vi "PCert-ConfigPageNF-AskDB.vi"(6 "Timeout":i32=100 format="%dmsec", 8 "error in (no error)":errorcluster, 9 "Request Body":string, 10 "Request Header":string, 11 "ERP-ConfigPageNF in":refnum<class "PCert-ConfigPageNF.lvclass">) -> (0 "error out":errorcluster, 2 "Ask Operation Failed":bool, 3 "ERP-ConfigPageNF out":refnum<class "PCert-ConfigPageNF.lvclass">, 5 "Raw Column Data From DB":string[](array[string]), 7 "Raw Data From DB":string[][](array[string]))   [LabVIEW 2013, in "PCert-ConfigPageNF.lvclass"]
uses:
  PCert-ConfigPageNF.lvclass
  PCert-ConfigPageNF.lvclass/PCert-ConfigPageNF.ctl
  ftw-dataflow/Actor/src/Connector/FTW-ActorConnector.lvclass
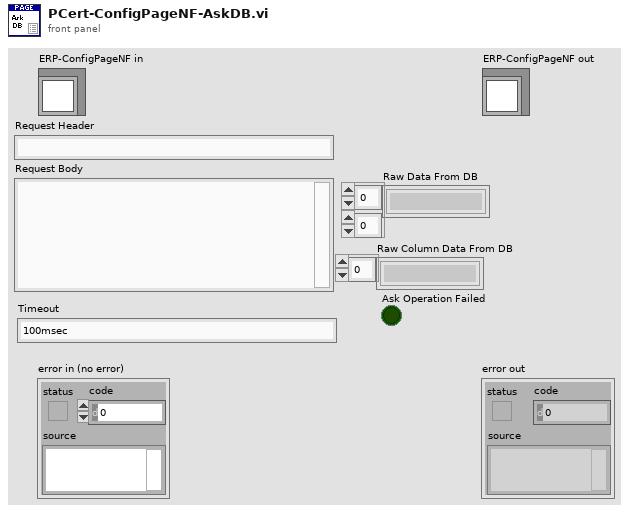
[diagram p1: front panel]
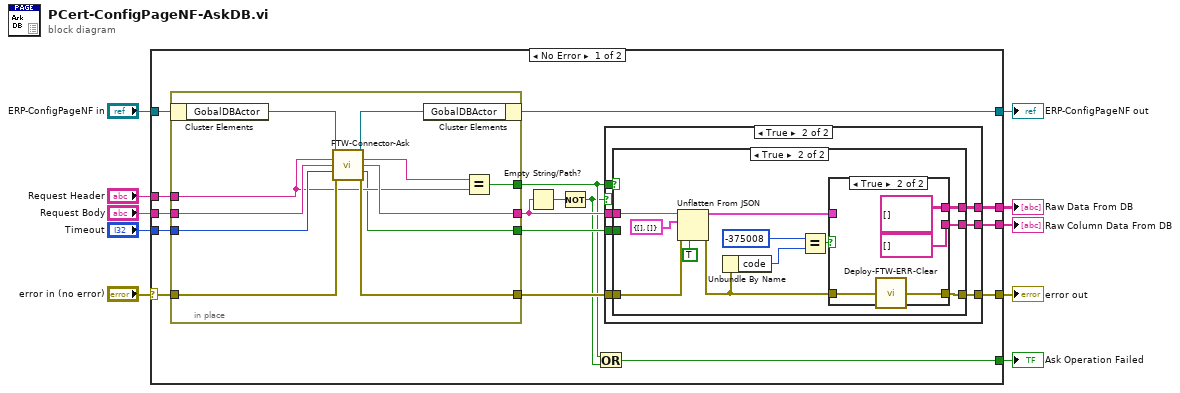
[diagram p0: block diagram]
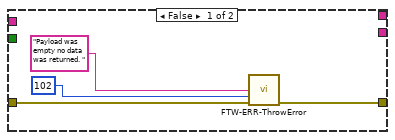
[diagram p2: hidden frame]
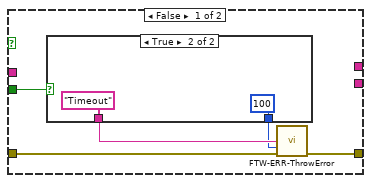
[diagram p3: hidden frame]
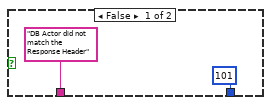
[diagram p4: hidden frame]
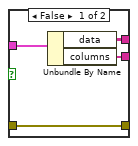
[diagram p5: hidden frame]
diagram:
  n1 = case shown="No Error" "error in (no error)" {
    selector: "error in (no error)" -> [w25 w79]
    tunnel: [w19 w79] -> w9
    tunnel: [w21 w78] -> w7
    tunnel: "ERP-ConfigPageNF in" -> [w26 w78]
    tunnel: "Request Header" -> [w24 _]
    tunnel: "Request Body" -> [w23 _]
    tunnel: "Timeout" -> [w22 _]
    tunnel: [w18 _] -> w3
    tunnel: [w17 _] -> w2
    tunnel: [w11 _] -> w1
    frame No Error {
      n2 = in-place {
        in-place-border: w25 -> [w75]
        in-place-border: [w74] -> w20
        in-place-border: w24 -> [w69]
        in-place-border: w23 -> [w73]
        in-place-border: w22 -> [w72]
        in-place-border: [w71] -> w15
        in-place-border: [w68] -> w13
        in-place-border: [w67] -> w16
        n3 = in-place-cluster #1(w26) -> ("GobalDBActor"=w77:refnum<class "FTW-ActorConnector.lvclass">)
        n4 = call "FTW-Connector-Ask.vi"("FTW Actor Connector"=w77, "Request Header"=w69, "Request Body"=w73, "Timeout"=w72, "error in"=w75) -> ("FTW Actor Connector out"=w76:refnum<class "FTW-ActorConnector.lvclass">, "Response Header"=w70:string, "Response Body"=w71:string, "Timed out?"=w67:bool, "error out"=w74:errorcluster)  [unwired: 6 in]
        n5 = in-place-cluster #1("GobalDBActor"=w76) -> (w21:refnum<class "PCert-ConfigPageNF.lvclass">)
        n6 = Equal?(x=w70, y=w69) -> (x = y?=w68:bool)
      }
      n7 = Empty String/Path?(string/path=w15) -> (empty?=w14:bool)
      n8 = Not(x=w14) -> (.not. x?=w12:bool)
      n9 = Or(x=w13, y=w12) -> (x .or. y?=w11:bool)
      n10 = case shown="True" w12 {
        tunnel: w13 -> [_ w37]
        tunnel: w20 -> [w30 w36]
        tunnel: [w27 w35] -> w19
        tunnel: [_ w34] -> w18
        tunnel: [_ w33] -> w17
        tunnel: w16 -> [_ w32]
        tunnel: w15 -> [_ w31]
        frame False {
          n11 = call "FTW-ERR-ThrowError.vi"("Error Message"="Payload was empty no data was returned. " ("source"), "Error Code"=102, "error in"=w30) -> ("error out"=w27:errorcluster)  [unwired: 12 in]
        }
        frame True {
          n12 = case shown="True" w37 {
            tunnel: w36 -> [w42 w56]
            tunnel: w31 -> [_ w53]
            tunnel: [w40 w47] -> w35
            tunnel: [_ w58] -> w34
            tunnel: [_ w57] -> w33
            tunnel: w32 -> [w38 _]
            frame False {
              n13 = case shown="True" w38 {
                tunnel: ["DB Actor did not match the Response Header" ("source") "Timeout" ("source")] -> w41
                tunnel: [101 ("Error Code") 100 ("Error Code")] -> w39
                frame False {
                }
                frame True {
                }
              }
              n14 = call "FTW-ERR-ThrowError.vi"("Error Message"=w41, "Error Code"=w39, "error in"=w42) -> ("error out"=w40:errorcluster)  [unwired: 12 in]
            }
            frame True {
              n15 = Unflatten From JSON(JSON string=w53, type and defaults=cluster{"data":string[][], "columns":string[]} {"data"=[], "columns"=[]}, default null elements? (F)=TRUE, error in (no error)=w56) -> (value=w54:cluster{"data":string[][], "columns":string[]}, error out=w48:errorcluster)  [unwired: 3 in]
              n16 = Unbundle By Name(w48) -> ("code"=w51:i32)
              n17 = Equal?(x=-375008, y=w51) -> (x = y?=w49:bool)
              n18 = case shown="True" w49 {
                tunnel: [w62 string[][] [] ("data")] -> w58
                tunnel: [w61 string[] [] ("columns")] -> w57
                tunnel: w54 -> [w60 _]
                tunnel: w48 -> [w59 w66]
                tunnel: [w59 w65] -> w47
                frame False {
                  n19 = Unbundle By Name(w60) -> ("data"=w62:string[][], "columns"=w61:string[])
                }
                frame True {
                  n20 = call <resource>:"Deploy-FTW-ERR-Clear.vi"("error to snuff"=w66) -> ("no error"=w65:errorcluster)
                }
              }
            }
          }
        }
      }
    }
    frame Error {
    }
  }
  "error out" <- w9
  "ERP-ConfigPageNF out" <- w7
  "Raw Data From DB" <- w3
  "Raw Column Data From DB" <- w2
  "Ask Operation Failed" <- w1
